vi "Select_Strings.vi"(4 "Timeout (s)":dbl=nan, 5 "Available Ch names":string[](array[string]), 6 "Message":string, 7 "Selector mode":T1(ring), 8 "Desired Ch names (in)":string[](array[string])) -> (0 "Ch Indicies Chosen":i32[](array[numeric]), 1 "Cancel":bool, 2 "Selected Channel Names":string[](array[string]))   [LabVIEW 2022 SP3]
panel:
  out "Auto-dismiss":dbl(slide) scale=0.0..60.0
  in  "Cancel 1":bool
  in  "OK":bool
  in  "Search String":string
  in  "Selector":i32[](listbox)
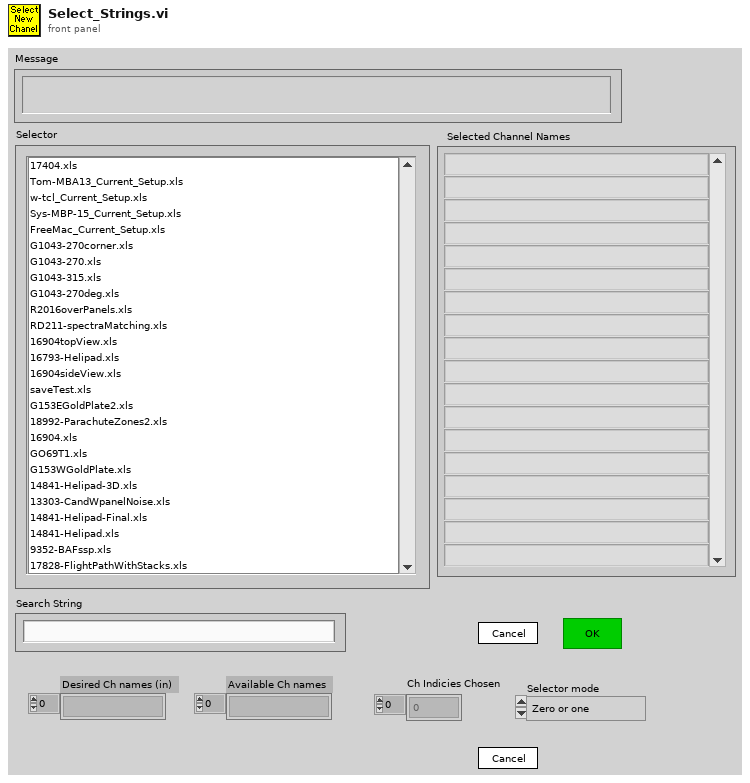
[diagram p1: front panel]
types:
  T1 = enum16{"Zero or one", "One", "Zero or more", "One or more"}
  T2 = enum8{"Enabled", "Disabled", "Disabled and Grayed Out"}
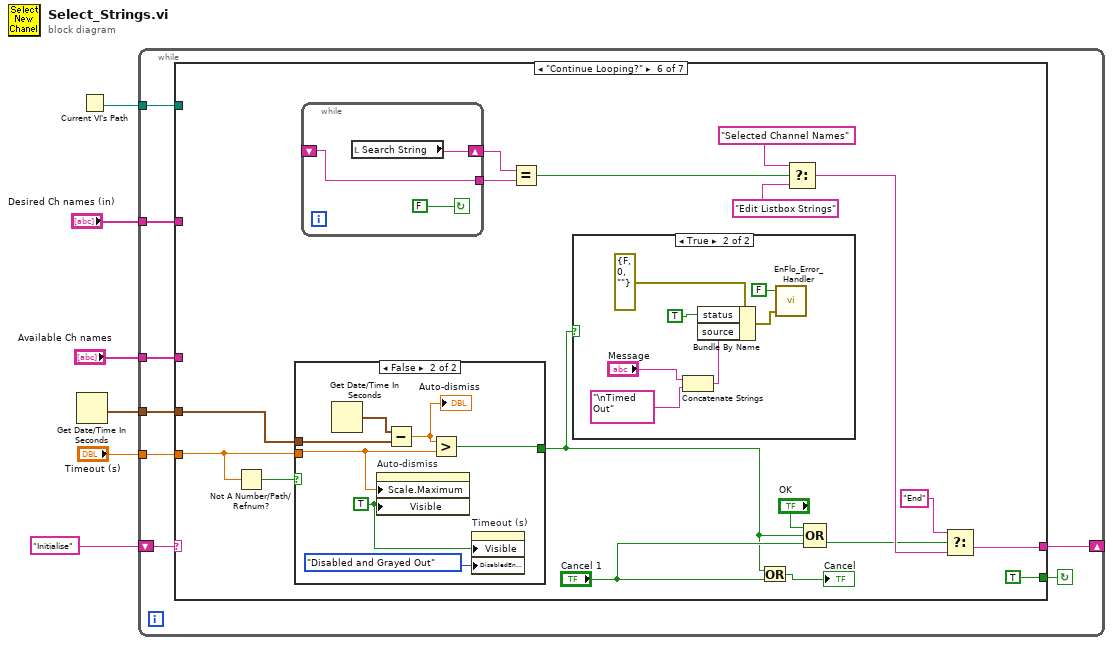
[diagram p0: block diagram]
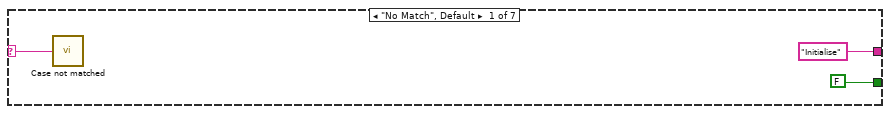
[diagram p2: hidden frame]
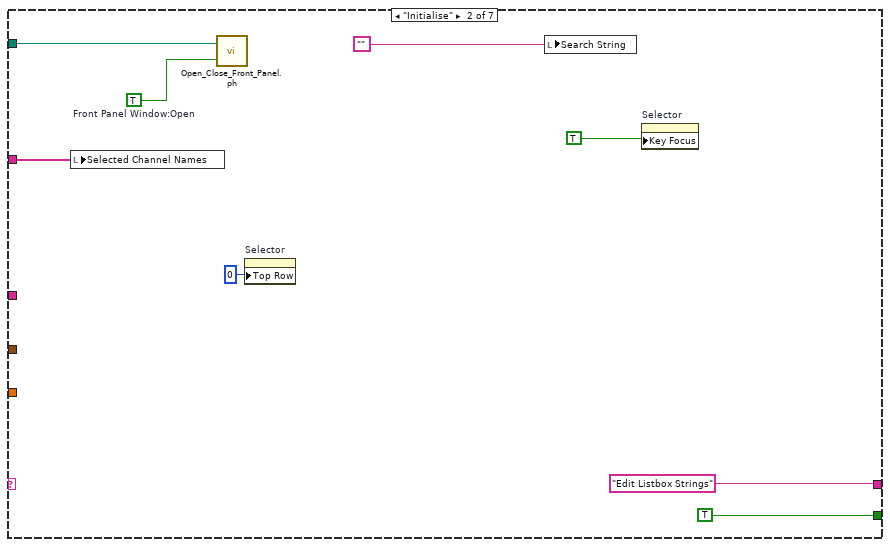
[diagram p3: hidden frame]
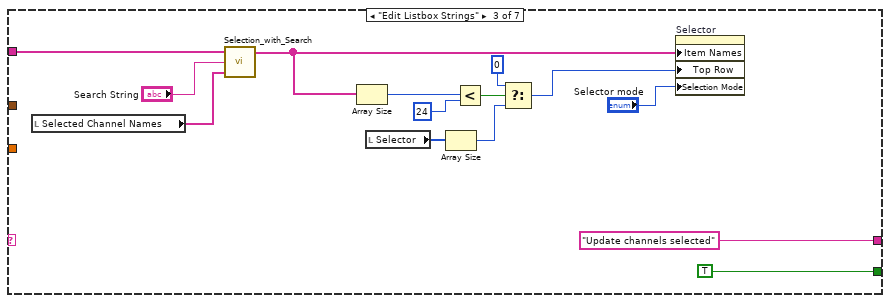
[diagram p4: hidden frame]
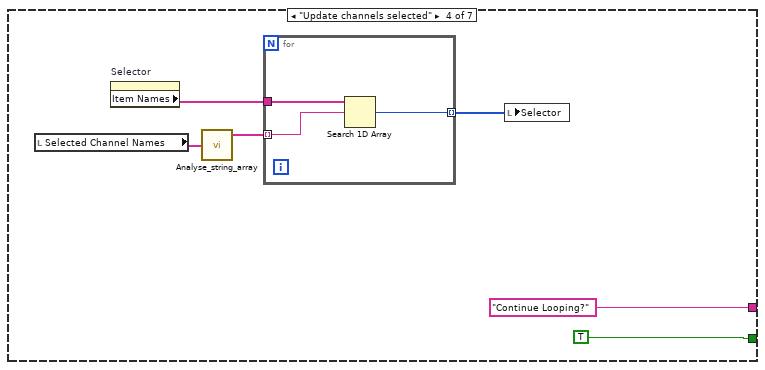
[diagram p5: hidden frame]
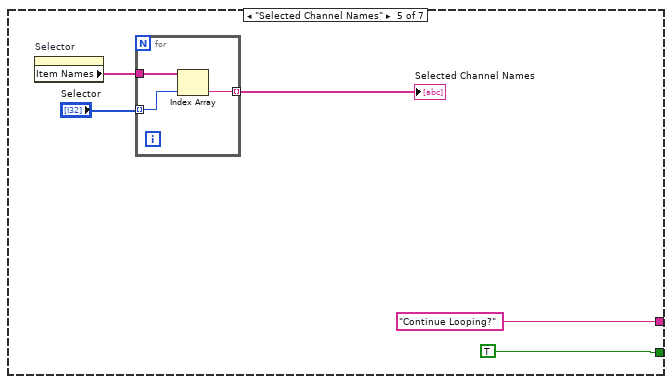
[diagram p6: hidden frame]
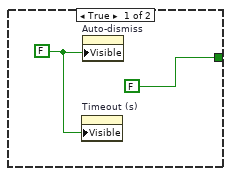
[diagram p8: hidden frame]
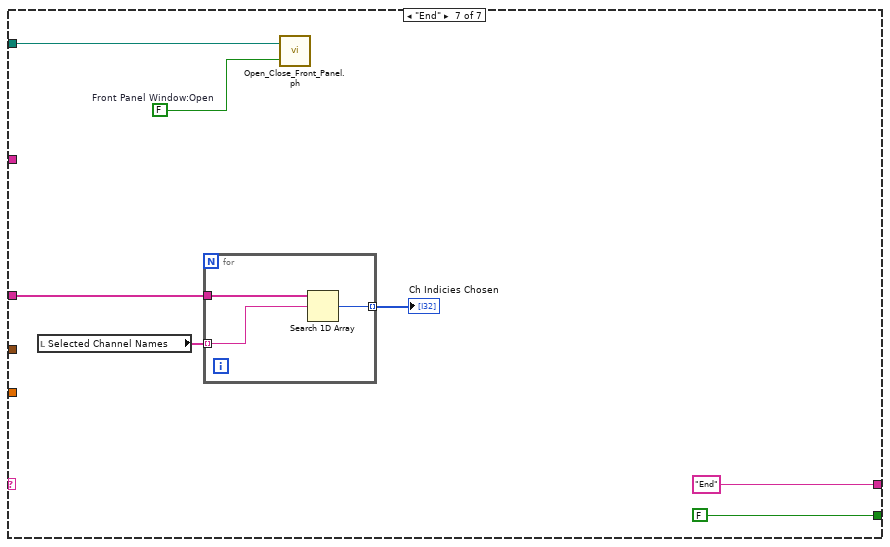
[diagram p9: hidden frame]
diagram:
  n1 = Get Date/Time In Seconds() -> (seconds since 1Jan1904=w2:timestamp)
  n2 = Current VI's Path() -> (path=w3:path)
  n3 = while {
    shift-left: "Initialise" -> [w12]
    shift-right: [w13] -> _
    tunnel: "Desired Ch names (in)" -> [w11]
    tunnel: "Available Ch names" -> [w10]
    tunnel: w3 -> [w9]
    tunnel: w2 -> [w8]
    tunnel: "Timeout (s)" -> [w7]
    stop <- w14 continue-if-true
    n4 = case shown="\"Continue Looping?\"" w12 {
      selector: w12 -> [w15 _ _ _ _ _ _]
      tunnel: [FALSE TRUE TRUE TRUE TRUE TRUE FALSE] -> w14
      tunnel: ["Initialise" "Edit Listbox Strings" "Update channels selected" "Continue Looping?" "Continue Looping?" w67 "End" ("t")] -> w13
      tunnel: w11 -> [_ w19 _ _ _ _ _]
      tunnel: w10 -> [_ _ w35 _ _ _ w97]
      tunnel: w9 -> [_ w23 _ _ _ _ w94]
      tunnel: w8 -> [_ _ _ _ _ w63 _]
      tunnel: w7 -> [_ _ _ _ _ w61 _]
      frame "No Match", Default {
        n5 = call "Case not matched.vi"("Case Name not Matched"=w15) -> ()
      }
      frame "Initialise" {
        w22 = TRUE  # Front Panel Window:Open
        n6 = local write "Selected Channel Names"(w19) -> ()
        n7 = call "Open_Close_Front_Panel.ph.vi"("openWindow (T)"=w22, "VI path"=w23) -> ()  [unwired: 1 in, 1 out]
        n8 = property on="Selector" class="LstBox (strict)"("Top Row"=0) -> ()  [unwired: 2 in, 2 out]
        n9 = local write "Search String"("") -> ()
        n10 = property on="Selector" class="LstBox (strict)"("Key Focus"=TRUE) -> ()  [unwired: 2 in, 2 out]
      }
      frame "Edit Listbox Strings" {
        n11 = local read "Selected Channel Names"() -> (w36:string[])
        n12 = call "Selection_with_Search.vi"("Selected Channel Names"=w36, "Search String"="Search String", "All Channel Names"=w35) -> ("Item Names"=w28:string[])
        n13 = Array Size(array=w28) -> (size(s)=w33:i32)
        n14 = local read "Selector"() -> (w27:i32[])
        n15 = Array Size(array=w27) -> (size(s)=w26:i32)
        n16 = Less?(x=w33, y=24) -> (x < y?=w32:bool)
        n17 = Select(t=0, s=w32, f=w26) -> (s? t:f=w31:i32)
        n18 = property on="Selector" class="LstBox (strict)"("Item Names"=w28, "Top Row"=w31, "Selection Mode"="Selector mode") -> ()  [unwired: 2 in, 2 out]
      }
      frame "Update channels selected" {
        n19 = local read "Selected Channel Names"() -> (w41:string[])
        n20 = property on="Selector" class="LstBox (strict)"() -> ("Item Names"=w43:string[])  [unwired: 2 in, 2 out]
        n21 = call "Analyse_string_array.vi"("String array"=w41) -> ("Unique strings"=w40:string[])  [unwired: 1 in, 1 out]
        n22 = for {
          tunnel: w43 -> [w48]
          tunnel: w40 -> [w47] mode=indexing
          tunnel: [w46] -> w42 mode=indexing
          n23 = Search 1D Array(1D array=w48, element=w47) -> (index of element=w46:i32)  [unwired: 1 out]
        }
        n24 = local write "Selector"(w42) -> ()
      }
      frame "Selected Channel Names" {
        n25 = property on="Selector" class="LstBox (strict)"() -> ("Item Names"=w51:string[])  [unwired: 2 in, 2 out]
        n26 = for {
          tunnel: w51 -> [w56]
          tunnel: "Selector" -> [w55] mode=indexing
          tunnel: [w54] -> w49 mode=indexing
          n27 = Index Array(array=w56, index=w55) -> (element=w54:string)
        }
        "Selected Channel Names" <- w49
      }
      frame "Continue Looping?" {
        n28 = Not A Number/Path/Refnum?(number/path/refnum=w61) -> (NaN/Path/Refnum?=w62:bool)
        n29 = case shown="False" w62 {
          tunnel: w63 -> [_ w88]
          tunnel: w61 -> [_ w85]
          tunnel: [FALSE w87] -> w58
          frame True {
            w81 = FALSE ("Visible")
            n30 = property on="Timeout (s)" class="DigNum (strict)"("Visible"=w81) -> ()  [unwired: 2 in, 2 out]
            n31 = property on="Auto-dismiss" class="Slide (strict)"("Visible"=w81) -> ()  [unwired: 2 in, 2 out]
          }
          frame False {
            w84 = TRUE ("Visible")
            n32 = Get Date/Time In Seconds() -> (seconds since 1Jan1904=w89:timestamp)
            n33 = property on="Auto-dismiss" class="Slide (strict)"("Scale.Maximum"=w85, "Visible"=w84) -> ()  [unwired: 2 in, 2 out]
            n34 = Subtract(x=w89, y=w88) -> (x-y=w86:dbl)
            "Auto-dismiss" <- w86
            n35 = Greater?(x=w86, y=w85) -> (0:w87:bool)
            n36 = property on="Timeout (s)" class="DigNum (strict)"("Visible"=w84, "DisabledEnum"=T2."Disabled and Grayed Out" ("Disabled")) -> ()  [unwired: 2 in, 2 out]
          }
        }
        n37 = while {
          tunnel: [w91] -> w73
          shift-left: _ -> [w91]
          shift-right: [w92] -> w72
          stop <- FALSE continue-if-true
          n38 = local read "Search String"() -> (w92:string)
        }
        n39 = Equal?(x=w72, y=w73) -> (x = y?=w71:bool)
        n40 = case shown="True" w58 {
          frame False {
          }
          frame True {
            n41 = Concatenate Strings("Message", "\nTimed Out" ("string")) -> (w75:string)
            n42 = Bundle By Name(cluster=errorcluster {"status"=FALSE, "code"=0, "source"=""} ("error in (no error)"), "status"=TRUE, "source"=w75) -> (w77:errorcluster)
            n43 = call "EnFlo_Error_Handler.vi"("error in (no error)"=w77, "Dialog Box (F)"=FALSE ("Dialog Box (T)")) -> ()  [unwired: 2 in, 2 out]
          }
        }
        n44 = Or(x=w58, y="Cancel 1") -> (x .or. y?=→"Cancel":bool)
        n45 = Select(t="Selected Channel Names", s=w71, f="Edit Listbox Strings") -> (s? t:f=w66:string)
        n46 = Compound Arithmetic op=OR("OK", w58, "Cancel 1") -> (w64:bool)
        n47 = Select(t="End", s=w64, f=w66) -> (s? t:f=w67:string)
      }
      frame "End" {
        w93 = FALSE  # Front Panel Window:Open
        n48 = local read "Selected Channel Names"() -> (w96:string[])
        n49 = for {
          tunnel: w97 -> [w102]
          tunnel: w96 -> [w101] mode=indexing
          tunnel: [w100] -> w95 mode=indexing
          n50 = Search 1D Array(1D array=w102, element=w101) -> (index of element=w100:i32)  [unwired: 1 out]
        }
        "Ch Indicies Chosen" <- w95
        n51 = call "Open_Close_Front_Panel.ph.vi"("openWindow (T)"=w93, "VI path"=w94) -> ()  [unwired: 1 in, 1 out]
      }
    }
  }
